vi "Close Serial.vi"(8 "error in (no error)":errorcluster, 11 "VISA Reference":refnum<visa-resource-name>) -> (0 "error out":errorcluster)   [LabVIEW 2019, in "PGC2D.lvlib"]
uses:
  PGC2D.lvlib
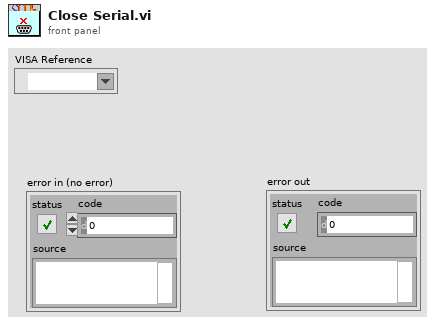
[diagram p1: front panel]
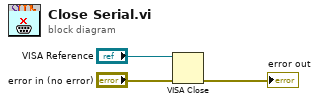
[diagram p0: block diagram]
diagram:
  n1 = VISA Close(VISA resource name="VISA Reference", error in (no error)="error in (no error)") -> (error out=→"error out":errorcluster)
